vi "CTRE_Phoenix_CANcoder_GetLastUnitString.vi"(0 "CTRE_CANcoder_DeviceRef":T1, 11 "error in":errorcluster) -> (4 "CTRE_CANcoder_DeviceRef":T1, 6 "unitString":string, 15 "error out":errorcluster)   [LabVIEW 2020]
doc: "Get the units for the signal retrieved in the last called get routine."
uses:
  <vilib>/Rock Robotics/WPI/ThirdParty/Phoenix-LabVIEW/CANCoder/Controls/CTRE_Phoenix_CANcoder_DeviceRef.ctl
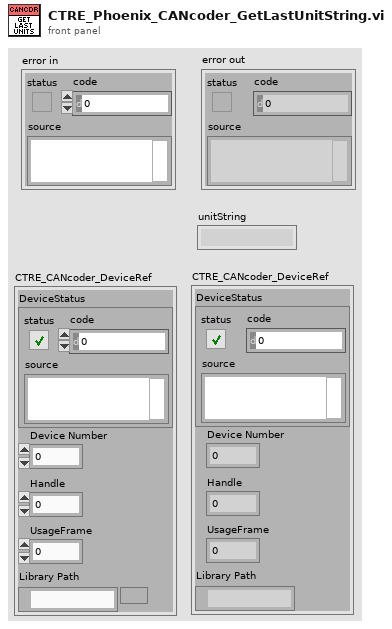
[diagram p1: front panel]
types:
  T1 = typedef "CTRE_Phoenix_CANcoder_DeviceRef.ctl" = cluster{"DeviceStatus":errorcluster, "Device Number":u8, "Handle":u64, "UsageFrame":u32, "Library Path":path}
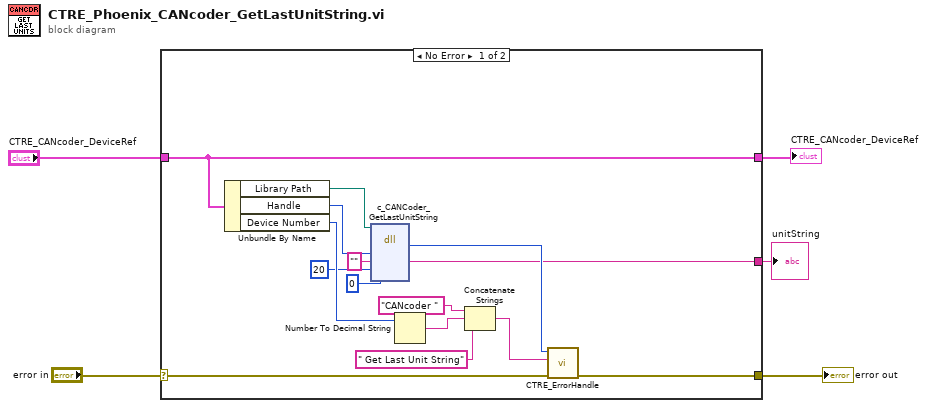
[diagram p0: block diagram]
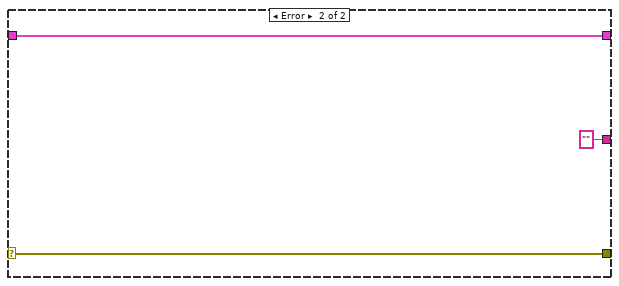
[diagram p2: hidden frame]
diagram:
  n1 = case shown="No Error" "error in" {
    selector: "error in" -> [w17 w23]
    tunnel: "CTRE_CANcoder_DeviceRef" -> [w18 w22]
    tunnel: [w16 w23] -> w4
    tunnel: [w18 w22] -> w2
    tunnel: [w6 "" ("unitString")] -> w1
    frame No Error {
      n2 = Unbundle By Name(w18) -> ("Library Path"=w20:path, "Handle"=w19:u64, "Device Number"=w10:u8)
      n3 = dll-call lib="?" fn="c_CANCoder_GetLastUnitString"(path in=w20, "handle"=w19, "unitString"="", "toFillByteSz"=20, "numBytesFilled"=0) -> ("CTR_Code"=w15:i8, "unitString"=w6:string)  [unwired: 5 in, 2 out]
      n4 = Number To Decimal String(number=w10) -> (decimal integer string=w14:string)  [unwired: 1 in]
      n5 = Concatenate Strings("CANcoder " ("string"), w14, " Get Last Unit String" ("string")) -> (w11:string)
      n6 = call <vilib>:"CTRE_ErrorHandle.vi"("error in"=w17, "origin"=w11, "code"=w15) -> ("error out"=w16:errorcluster)  [unwired: 8 in]
    }
    frame Error {
    }
  }
  "error out" <- w4
  "CTRE_CANcoder_DeviceRef" <- w2
  "unitString" <- w1
